vi "Read Port.vi"(8 "error in (no error)":errorcluster, 11 "Socket Communication in":refnum<class "Socket Communication.lvclass">) -> (0 "error out":errorcluster, 2 "Port":u16, 3 "Socket Communication out":refnum<class "Socket Communication.lvclass">)   [LabVIEW 2019, in "Socket Communication.lvclass"]
uses:
  Socket Communication.lvclass
  Socket Communication.lvclass/Socket Communication.ctl
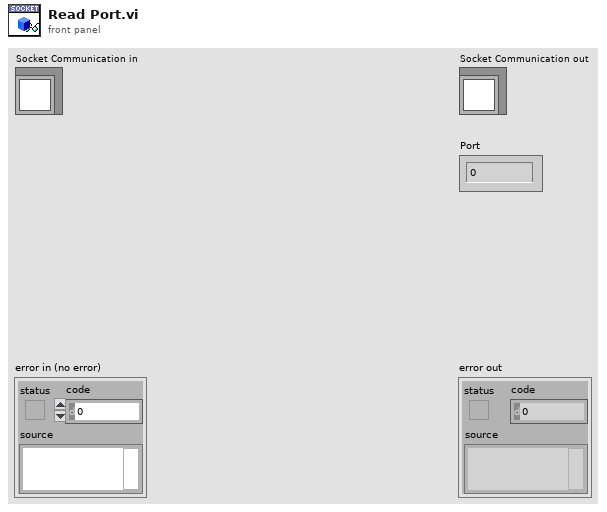
[diagram p1: front panel]
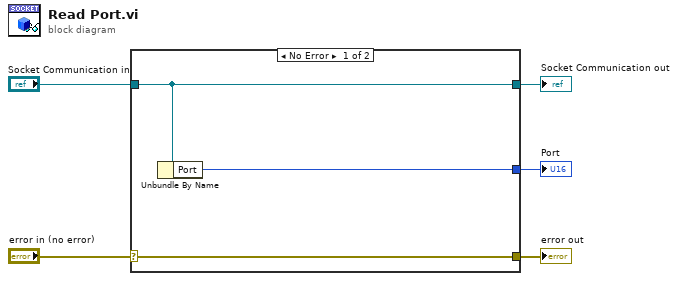
[diagram p0: block diagram]
diagram:
  n1 = case shown="No Error" "error in (no error)" {
    selector: "error in (no error)" -> [w8 w9]
    tunnel: [w8 w9] -> w4
    tunnel: [w7 w10] -> w2
    tunnel: "Socket Communication in" -> [w7 w10]
    tunnel: [w6 _] -> w1
    frame No Error {
      n2 = Unbundle By Name(w7) -> ("Port"=w6:u16)
    }
    frame Error {
    }
  }
  "error out" <- w4
  "Socket Communication out" <- w2
  "Port" <- w1
